vi "button commands.vi"(6 "Configuration":T1, 7 "Z Steps":dbl, 8 "Motion":T2, 9 "Y Steps":dbl, 10 "mapped gp buttons":T3, 11 "X Steps":dbl) -> (0 "Y distance":dbl, 1 "Choose Button":bool, 2 "Z distance":dbl, 3 "X distance":dbl)   [LabVIEW 2012]
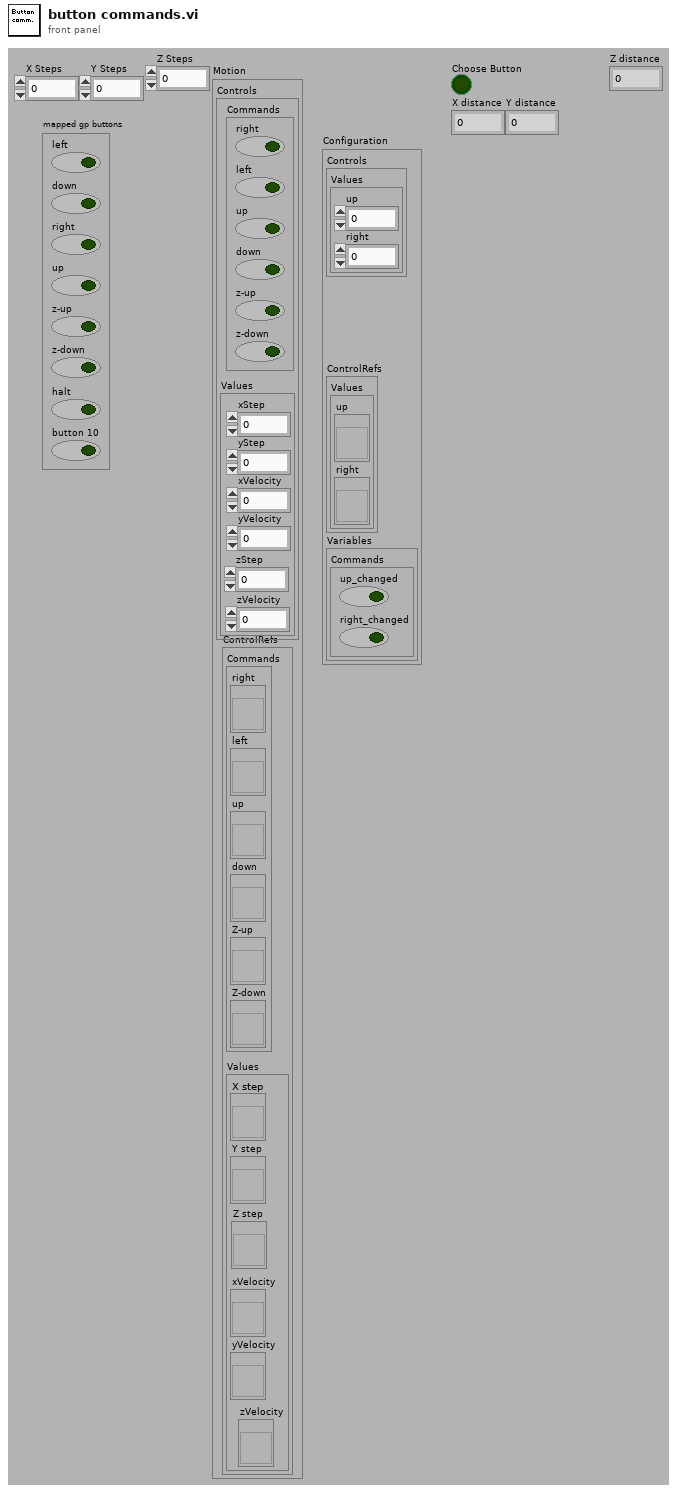
[diagram p1: front panel]
types:
  T1 = cluster{"Controls":cluster{"Values":cluster{"up":u16, "right":u16}}, "ControlRefs":cluster{"Values":cluster{"up":refnum<vi>, "right":refnum<vi>}}, "Variables":cluster{"Commands":cluster{"up_changed":bool, "right_changed":bool}}}
  T2 = cluster{"Controls":cluster{"Commands":cluster{"right":bool, "left":bool, "up":bool, "down":bool, "z-up":bool, "z-down":bool}, "Values":cluster{"xStep":dbl, "yStep":dbl, "xVelocity":dbl, "yVelocity":dbl, "zStep":dbl, "zVelocity":dbl}}, "ControlRefs":cluster{"Commands":cluster{"right":refnum<vi>, "left":refnum<vi>, "up":refnum<vi>, "down":refnum<vi>, "Z-up":refnum<vi>, "Z-down":refnum<vi>}, "Values":cluster{"X step":refnum<vi>, "Y step":refnum<vi>, "xVelocity":refnum<vi>, "yVelocity":refnum<vi>, "Z step":refnum<vi>, "zVelocity":refnum<vi>}}}
  T3 = cluster{"left":bool, "down":bool, "right":bool, "up":bool, "z-up":bool, "z-down":bool, "halt":bool, "button 10":bool}
  T4 = cluster{"xf":bool, "xr":bool, "yf":bool, "yr":bool, "zf":bool, "zr":bool}
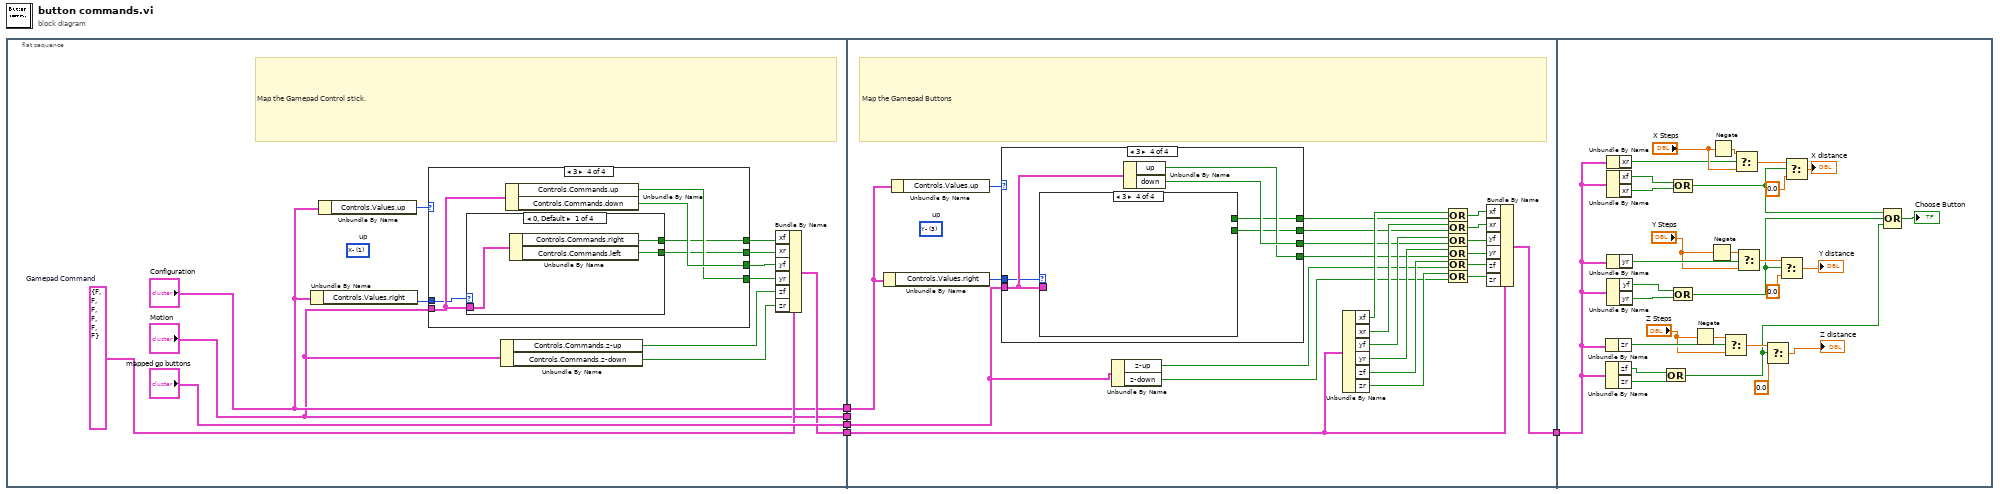
[diagram p0: block diagram]
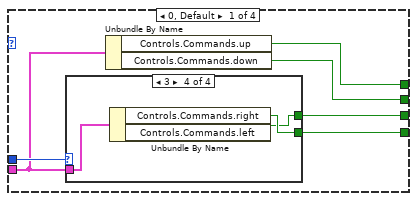
[diagram p2: hidden frame]
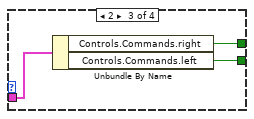
[diagram p5: hidden frame]
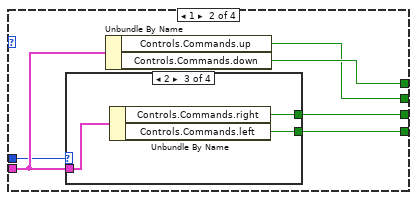
[diagram p6: hidden frame]
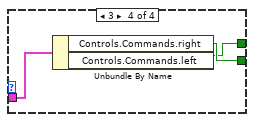
[diagram p9: hidden frame]
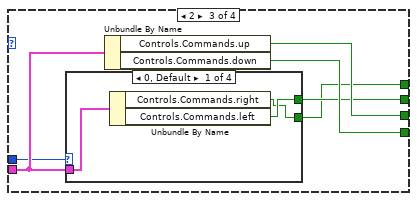
[diagram p10: hidden frame]
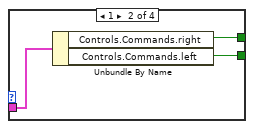
[diagram p11: hidden frame]
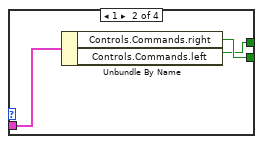
[diagram p14: hidden frame]
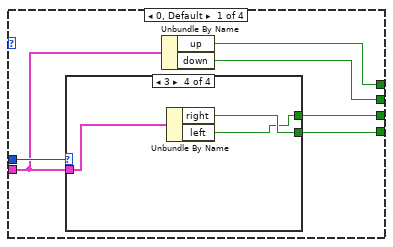
[diagram p17: hidden frame]
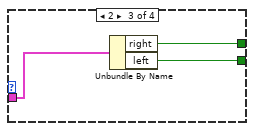
[diagram p20: hidden frame]
diagram:
  n1 = flat-sequence {
    tunnel: ["mapped gp buttons"] -> w4
    tunnel: [w16] -> w3
    tunnel: ["Motion"] -> w2
    tunnel: ["Configuration"] -> w1
    tunnel: w4 -> [w73]
    tunnel: w3 -> [w81]
    tunnel: [w87] -> w5
    tunnel: w2 -> [_]
    tunnel: w1 -> [w88]
    tunnel: w5 -> [w149]
    frame #0 {
      w17 = T4 {"xf"=FALSE, "xr"=FALSE, "yf"=FALSE, "yr"=FALSE, "zf"=FALSE, "zr"=FALSE}  # Gamepad Command
      (unwired) u16 1 items=["X+", "X-", "Y+", "Y-"]  # up
      # "Map the Gamepad Control stick."
      n2 = Unbundle By Name("Configuration") -> ("Controls.Values.right"=w13:u16)
      n3 = Unbundle By Name("Configuration") -> ("Controls.Values.up"=w15:u16)
      n4 = case shown="3" w15 {
        tunnel: [w24 w34 w43 w55] -> w14
        tunnel: "Motion" -> [w21 w36 w48 w60]
        tunnel: w13 -> [w23 w35 w47 w59]
        tunnel: [w22 w33 w44 w56] -> w12
        tunnel: [w20 w31 w46 w58] -> w11
        tunnel: [w19 w32 w45 w57] -> w10
        frame 0, Default {
          n5 = case shown="3" w23 {
            tunnel: w21 -> [_ _ w27 w30]
            tunnel: [_ _ w26 w28] -> w20
            tunnel: [_ _ w25 w29] -> w19
            frame 0, Default {
            }
            frame 1 {
            }
            frame 2 {
              n6 = Unbundle By Name(w27) -> ("Controls.Commands.right"=w26:bool, "Controls.Commands.left"=w25:bool)
            }
            frame 3 {
              n7 = Unbundle By Name(w30) -> ("Controls.Commands.right"=w29:bool, "Controls.Commands.left"=w28:bool)
            }
          }
          n8 = Unbundle By Name(w21) -> ("Controls.Commands.up"=w24:bool, "Controls.Commands.down"=w22:bool)
        }
        frame 1 {
          n9 = case shown="2" w35 {
            tunnel: w36 -> [_ _ w39 w42]
            tunnel: [_ _ w37 w41] -> w32
            tunnel: [_ _ w38 w40] -> w31
            frame 0, Default {
            }
            frame 1 {
            }
            frame 2 {
              n10 = Unbundle By Name(w39) -> ("Controls.Commands.right"=w38:bool, "Controls.Commands.left"=w37:bool)
            }
            frame 3 {
              n11 = Unbundle By Name(w42) -> ("Controls.Commands.right"=w41:bool, "Controls.Commands.left"=w40:bool)
            }
          }
          n12 = Unbundle By Name(w36) -> ("Controls.Commands.up"=w33:bool, "Controls.Commands.down"=w34:bool)
        }
        frame 2 {
          n13 = case shown="0, Default" w47 {
            tunnel: w48 -> [w51 w54 _ _]
            tunnel: [w50 w53 _ _] -> w44
            tunnel: [w49 w52 _ _] -> w43
            frame 0, Default {
              n14 = Unbundle By Name(w51) -> ("Controls.Commands.right"=w49:bool, "Controls.Commands.left"=w50:bool)
            }
            frame 1 {
              n15 = Unbundle By Name(w54) -> ("Controls.Commands.right"=w53:bool, "Controls.Commands.left"=w52:bool)
            }
            frame 2 {
            }
            frame 3 {
            }
          }
          n16 = Unbundle By Name(w48) -> ("Controls.Commands.up"=w46:bool, "Controls.Commands.down"=w45:bool)
        }
        frame 3 {
          n17 = case shown="0, Default" w59 {
            tunnel: w60 -> [w63 w66 _ _]
            tunnel: [w61 w65 _ _] -> w56
            tunnel: [w62 w64 _ _] -> w55
            frame 0, Default {
              n18 = Unbundle By Name(w63) -> ("Controls.Commands.right"=w62:bool, "Controls.Commands.left"=w61:bool)
            }
            frame 1 {
              n19 = Unbundle By Name(w66) -> ("Controls.Commands.right"=w65:bool, "Controls.Commands.left"=w64:bool)
            }
            frame 2 {
            }
            frame 3 {
            }
          }
          n20 = Unbundle By Name(w60) -> ("Controls.Commands.up"=w57:bool, "Controls.Commands.down"=w58:bool)
        }
      }
      n21 = Unbundle By Name("Motion") -> ("Controls.Commands.z-up"=w7:bool, "Controls.Commands.z-down"=w6:bool)
      n22 = Bundle By Name(cluster=w17, "xf"=w14, "xr"=w12, "yf"=w11, "yr"=w10, "zf"=w7, "zr"=w6) -> (w16:T4)
    }
    frame #1 {
      (unwired) u16 3 items=["X+", "X-", "Y+", "Y-"]  # up
      # "Map the Gamepad Buttons"
      n23 = Unbundle By Name(w88) -> ("Controls.Values.right"=w90:u16)
      n24 = Unbundle By Name(w88) -> ("Controls.Values.up"=w89:u16)
      n25 = case shown="3" w89 {
        tunnel: [w94 w106 w115 w127] -> w70
        tunnel: w73 -> [w95 w108 w120 w132]
        tunnel: w90 -> [w96 w107 w119 w131]
        tunnel: [w93 w105 w116 w128] -> w69
        tunnel: [w92 w103 w118 w130] -> w68
        tunnel: [w91 w104 w117 w129] -> w67
        frame 0, Default {
          n26 = case shown="3" w96 {
            tunnel: w95 -> [_ _ w99 w102]
            tunnel: [_ _ w98 w100] -> w92
            tunnel: [_ _ w97 w101] -> w91
            frame 0, Default {
            }
            frame 1 {
            }
            frame 2 {
              n27 = Unbundle By Name(w99) -> ("right"=w98:bool, "left"=w97:bool)
            }
            frame 3 {
              n28 = Unbundle By Name(w102) -> ("right"=w101:bool, "left"=w100:bool)
            }
          }
          n29 = Unbundle By Name(w95) -> ("up"=w94:bool, "down"=w93:bool)
        }
        frame 1 {
          n30 = case shown="3" w107 {
            tunnel: w108 -> [_ _ w111 w114]
            tunnel: [_ _ w109 w113] -> w104
            tunnel: [_ _ w110 w112] -> w103
            frame 0, Default {
            }
            frame 1 {
            }
            frame 2 {
              n31 = Unbundle By Name(w111) -> ("right"=w110:bool, "left"=w109:bool)
            }
            frame 3 {
              n32 = Unbundle By Name(w114) -> ("right"=w113:bool, "left"=w112:bool)
            }
          }
          n33 = Unbundle By Name(w108) -> ("up"=w105:bool, "down"=w106:bool)
        }
        frame 2 {
          n34 = case shown="3" w119 {
            tunnel: w120 -> [w123 w126 _ _]
            tunnel: [w122 w125 _ _] -> w116
            tunnel: [w121 w124 _ _] -> w115
            frame 0, Default {
              n35 = Unbundle By Name(w123) -> ("right"=w121:bool, "left"=w122:bool)
            }
            frame 1 {
              n36 = Unbundle By Name(w126) -> ("right"=w125:bool, "left"=w124:bool)
            }
            frame 2 {
            }
            frame 3 {
            }
          }
          n37 = Unbundle By Name(w120) -> ("up"=w118:bool, "down"=w117:bool)
        }
        frame 3 {
          n38 = case shown="3" w131 {
            tunnel: w132 -> [w135 w136 _ _]
            tunnel: [w133 w138 _ _] -> w128
            tunnel: [w134 w137 _ _] -> w127
            frame 0, Default {
              n39 = Unbundle By Name(w135) -> ("right"=w134:bool, "left"=w133:bool)
            }
            frame 1 {
              n40 = Unbundle By Name(w136) -> ("right"=w138:bool, "left"=w137:bool)
            }
            frame 2 {
            }
            frame 3 {
            }
          }
          n41 = Unbundle By Name(w132) -> ("up"=w129:bool, "down"=w130:bool)
        }
      }
      n42 = Unbundle By Name(w73) -> ("z-up"=w72:bool, "z-down"=w71:bool)
      n43 = Unbundle By Name(w81) -> ("xf"=w79:bool, "xr"=w78:bool, "yf"=w77:bool, "yr"=w76:bool, "zf"=w75:bool, "zr"=w74:bool)
      n44 = Compound Arithmetic op=OR(w79, w70) -> (w86:bool)
      n45 = Compound Arithmetic op=OR(w78, w69) -> (w85:bool)
      n46 = Compound Arithmetic op=OR(w77, w68) -> (w84:bool)
      n47 = Compound Arithmetic op=OR(w76, w67) -> (w83:bool)
      n48 = Compound Arithmetic op=OR(w75, w72) -> (w82:bool)
      n49 = Compound Arithmetic op=OR(w74, w71) -> (w80:bool)
      n50 = Bundle By Name(cluster=w81, "xf"=w86, "xr"=w85, "yf"=w84, "yr"=w83, "zf"=w82, "zr"=w80) -> (w87:T4)
    }
    frame #2 {
      n51 = Unbundle By Name(w149) -> ("zr"=w146:bool)
      n52 = Unbundle By Name(w149) -> ("zf"=w148:bool, "zr"=w147:bool)
      n53 = Unbundle By Name(w149) -> ("xr"=w153:bool)
      n54 = Unbundle By Name(w149) -> ("xf"=w159:bool, "xr"=w160:bool)
      n55 = Unbundle By Name(w149) -> ("yr"=w151:bool)
      n56 = Unbundle By Name(w149) -> ("yf"=w157:bool, "yr"=w158:bool)
      n57 = Compound Arithmetic op=OR(w148, w147) -> (w139:bool)
      n58 = Compound Arithmetic op=OR(w159, w160) -> (w152:bool)
      n59 = Compound Arithmetic op=OR(w157, w158) -> (w140:bool)
      n60 = Negate(x="Z Steps") -> (-x=w145:dbl)
      n61 = Negate(x="Y Steps") -> (-x=w156:dbl)
      n62 = Negate(x="X Steps") -> (-x=w154:dbl)
      n63 = Select(t=w145, s=w146, f="Z Steps") -> (s? t:f=w144:dbl)
      n64 = Select(t=w154, s=w153, f="X Steps") -> (s? t:f=w163:dbl)
      n65 = Select(t=w156, s=w151, f="Y Steps") -> (s? t:f=w161:dbl)
      n66 = Select(t=w144, s=w139, f=0.0) -> (s? t:f=→"Z distance":dbl)
      n67 = Select(t=w161, s=w140, f=0.0) -> (s? t:f=→"Y distance":dbl)
      n68 = Select(t=w163, s=w152, f=0.0) -> (s? t:f=→"X distance":dbl)
      n69 = Compound Arithmetic op=OR(w152, w140, w139) -> (→"Choose Button":bool)
    }
  }
